vi "ErrorHandler_OBJ.vi"(7 "Mode":enum16{"Get", "Set"}(ring), 8 "error in":errorcluster, 11 "PROPERTIES IN":T1={"Log?"=TRUE, "DefaultAction"=enum."Clear", "actions"=[], "errorLog"=[], "writeLog?"=FALSE, "logPath"=path ""}) -> (0 "error out":errorcluster, 3 "PROPERTIES OUT":T1)   [LabVIEW 2013]
uses:
  ErrorHandler_OBJ - PROP.ctl
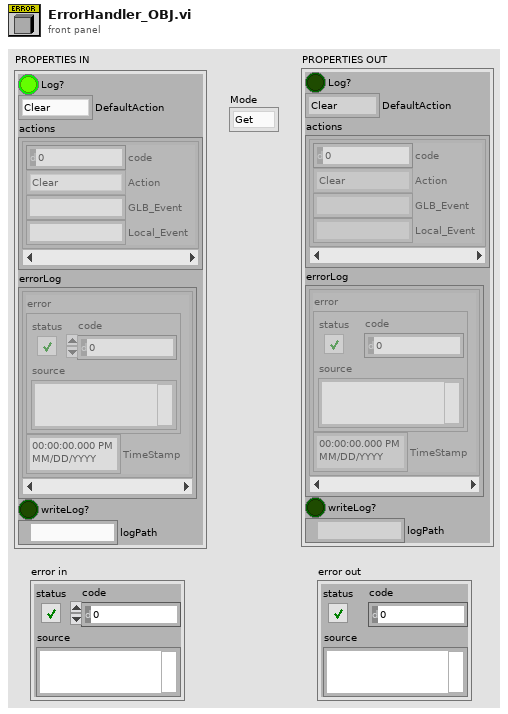
[diagram p1: front panel]
types:
  T1 = typedef "ErrorHandler_OBJ - PROP.ctl" = cluster{"Log?":bool, "DefaultAction":enum16{"Clear", "Continue"}, "actions":cluster{"code":i32, "Action":enum16{"Clear", "Continue"}, "GLB_Event":string, "Local_Event":string}[], "errorLog":cluster{"error":errorcluster, "TimeStamp":timestamp}[], "writeLog?":bool, "logPath":path}
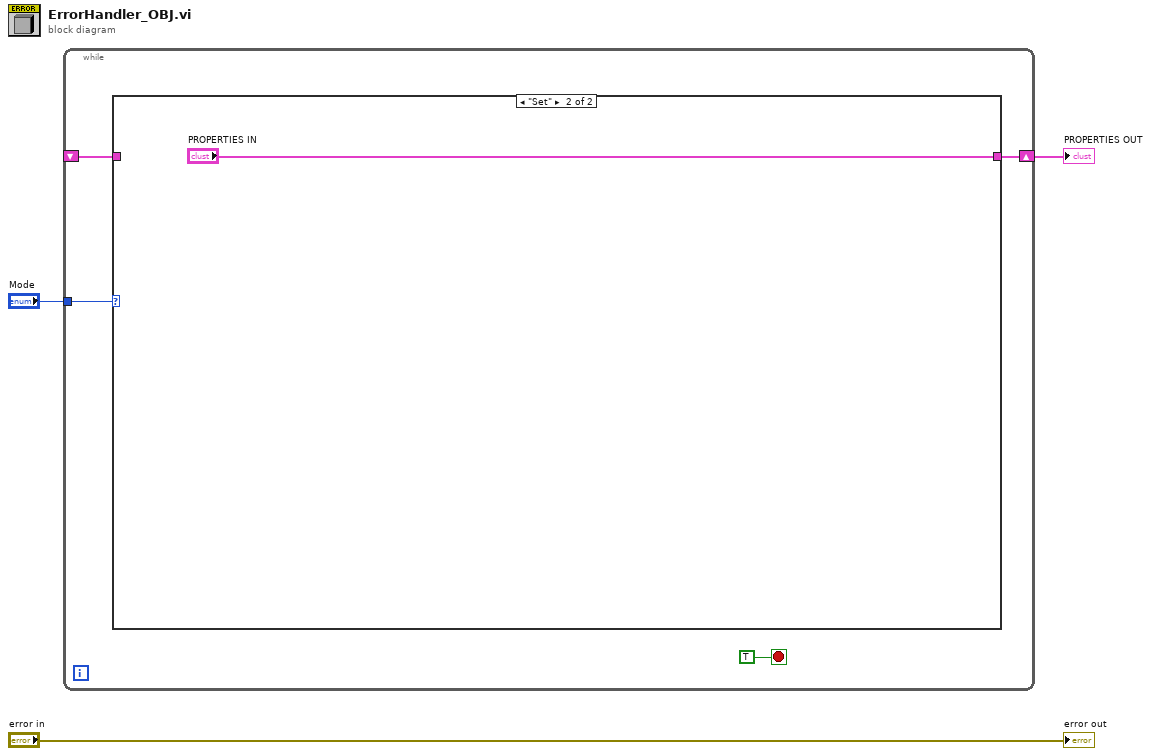
[diagram p0: block diagram]
diagram:
  n1 = while {
    tunnel: "Mode" -> [w6]
    shift-right: [w5] -> w2
    shift-left: _ -> [w4]
    stop <- TRUE stop-if-true
    n2 = case shown="\"Set\"" w6 {
      tunnel: [w8 "PROPERTIES IN"] -> w5
      tunnel: w4 -> [w8 _]
      frame "Get", Default {
      }
      frame "Set" {
      }
    }
  }
  "PROPERTIES OUT" <- w2
  "error out" <- "error in"
